vi "NavX SubVI _NEW.vi"(1 "error in (no error)":errorcluster) -> (2 "NavX Info Out":T2, 3 "NavX Output":T3, 4 "Timestamp":u32, 5 "error out":errorcluster)   [LabVIEW 2018]
uses:
  <vilib>/Studica/Studica Toolkit/Background/I2C Channel.ctl
  <vilib>/Studica/Studica Toolkit/NavX/NavX.lvlib
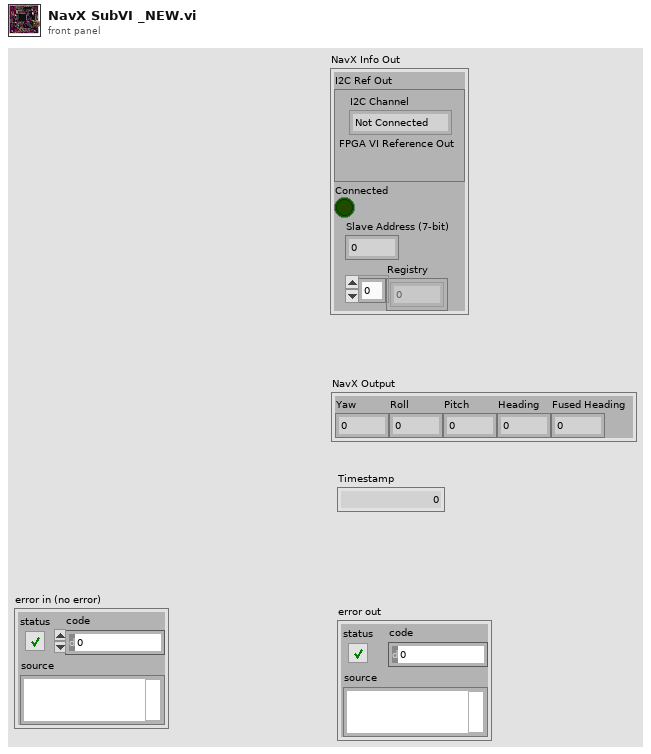
[diagram p1: front panel]
types:
  T1 = typedef "I2C Channel.ctl" = enum16{"Not Connected", "A", "B"}
  T2 = cluster{"I2C Ref Out":cluster{"I2C Channel":T1, "FPGA VI Reference Out":refnum<k20>}, "Connected":bool, "Slave Address (7-bit)":u8, "Registry":u8[]}
  T3 = cluster{"Yaw":dbl, "Roll":dbl, "Pitch":dbl, "Heading":dbl, "Fused Heading":dbl}
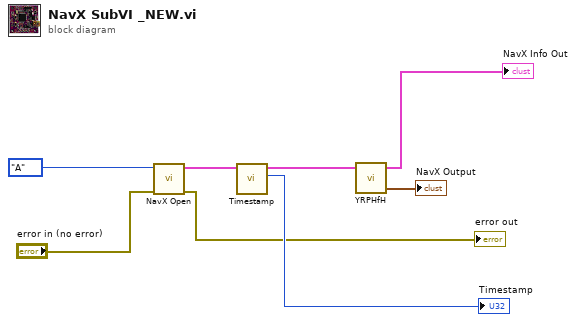
[diagram p0: block diagram]
diagram:
  n1 = call <vilib>:"NavX Open.vi"("error in (no error)"="error in (no error)", "I2C Channel"=I2C_Channel."A") -> ("error out"=→"error out":errorcluster, "NavX Info"=w6:T2)  [unwired: 8 in]
  n2 = call <vilib>:"Timestamp.vi"("NavX Info In"=w6) -> ("Timestamp"=→"Timestamp":u32, "NavX Info Out"=w2:T2)  [unwired: 9 in]
  n3 = call <vilib>:"YRPHfH.vi"("NavX Info In"=w2) -> ("YRPHfH"=→"NavX Output":T3, "NavX Info Out"=→"NavX Info Out":T2)  [unwired: 3 in]
